vi "Pcre2GetMatchDataOvector8.vi"(8 "error in":errorcluster, 9 "OvectorSize":u64, 11 "pMatchData":u64 format="%.0x") -> (0 "error out":errorcluster, 1 "MatchDataSize":u64, 2 "pOvector":u64 format="%.0x", 3 "pMatchData":u64 format="%.0x")   [LabVIEW 2021, in "libpcre2-8.lvlib"]
uses:
  libpcre2-8.lvlib
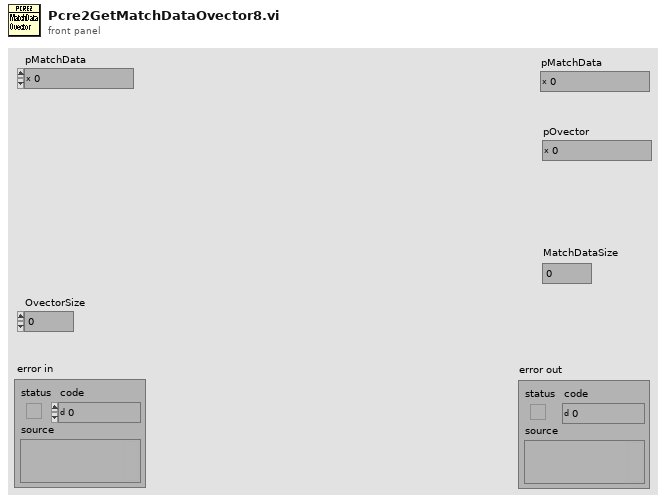
[diagram p1: front panel]
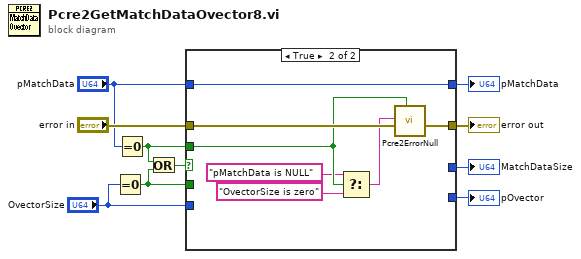
[diagram p0: block diagram]
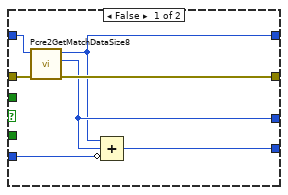
[diagram p2: hidden frame]
diagram:
  n1 = Equal To 0?(x="OvectorSize") -> (x = 0?=w3:bool)
  n2 = Equal To 0?(x="pMatchData") -> (x = 0?=w1:bool)
  n3 = Or(x=w1, y=w3) -> (x .or. y?=w4:bool)
  n4 = case shown="True" w4 {
    tunnel: "error in" -> [w15 w23]
    tunnel: [w14 w22] -> w9
    tunnel: "pMatchData" -> [w11 w24]
    tunnel: [w12 w24] -> w7
    tunnel: "OvectorSize" -> [w17 _]
    tunnel: [w16 _] -> w6
    tunnel: w3 -> [_ _]
    tunnel: [w13 _] -> w2
    tunnel: w1 -> [_ w20]
    frame False {
      n5 = call "Pcre2GetMatchDataSize8.vi"("error in"=w15, "pMatchData"=w11) -> ("error out"=w14:errorcluster, "MatchDataSize"=w13:u64, "pMatchData"=w12:u64)  [unwired: 7 in]
      n6 = Compound Arithmetic op=ADD(w12, w13, invert w17) -> (w16:u64)
    }
    frame True {
      n7 = Select(t="pMatchData is NULL" ("message"), s=w20, f="OvectorSize is zero" ("message")) -> (s? t:f=w21:string)
      n8 = call "Pcre2ErrorNull.vi"("IsPointer? (F)"=w20, "error in"=w23, "What"=w21) -> ("error out"=w22:errorcluster)  [unwired: 8 in]
    }
  }
  "pMatchData" <- w7
  "error out" <- w9
  "pOvector" <- w6
  "MatchDataSize" <- w2
